vi "PM100D_Single_Value_ph.vi"(2 "Averaging Period (s)":dbl=1.0, 3 "Beam Name":string="Green Unshifted") -> (0 "Status":T1, 1 "Light Power mW":dbl=8.10606551e-08 format="%^#_9e")   [LabVIEW 2012]
doc: "This VI shows how to communicate with a PM100D optical power/energy meter with SCPI commands.\n- Initializing the instrument\n- Getting system info\n- Setting parameters\n- Measurement configuration\n- Measuring queue\n- Fetching and displaying a measurement value\n- Closing the application"
uses:
  Gen Trav/Multi_Run_Status.ctl
panel:
  out "error out":errorcluster
  out "Wavelength nm":string="488"
  out "IDN String":string="Thorlabs,PM100USB,P2000214,1.3.0\n"
  out "Sensor SN":string="10020635"
  out "Sensor Name":string="S121C"
  out "Sensor Flags":bool[](array[boolean])=[TRUE, FALSE, FALSE, FALSE, FALSE, TRUE, FALSE, FALSE, TRUE, FALSE, FALSE, FALSE, FALSE, FALSE, FALSE, FALSE, FALSE, FALSE, FALSE, FALSE, FALSE, FALSE, FALSE, FALSE, FALSE, FALSE, FALSE, FALSE, FALSE, FALSE, FALSE, FALSE]
  out "New":bool=TRUE
  out "Timeout [ms]":i32=3000
  in  "Readout Config":string(combo)="POW"
  out "Readout string":string="81.06nW"
  out "Error log":string
  out "Averaging Rate":i32=2000
  # "1 Power Sensor"
  # "2 Energy Sensor"
  # "4"
  # "8"
  # "16 Response settable"
  # "32 Wavelength settable"
  # "64 Tau (time constant) settable"
  # "128"
  # "256 With temperature sensor"
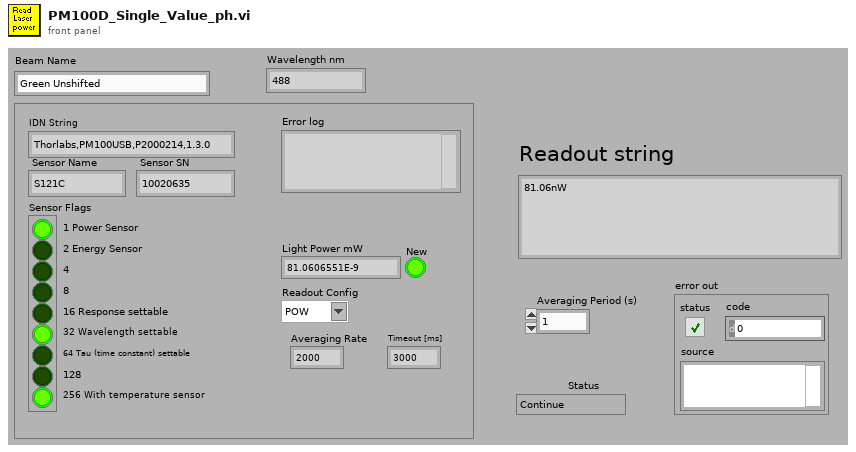
[diagram p1: front panel]
types:
  T1 = typedef "Multi_Run_Status.ctl" = enum16{"Continue", "Jump to Next Point", "Jump to Next Row", "Jump To Fall Back", "Terminate Run"}
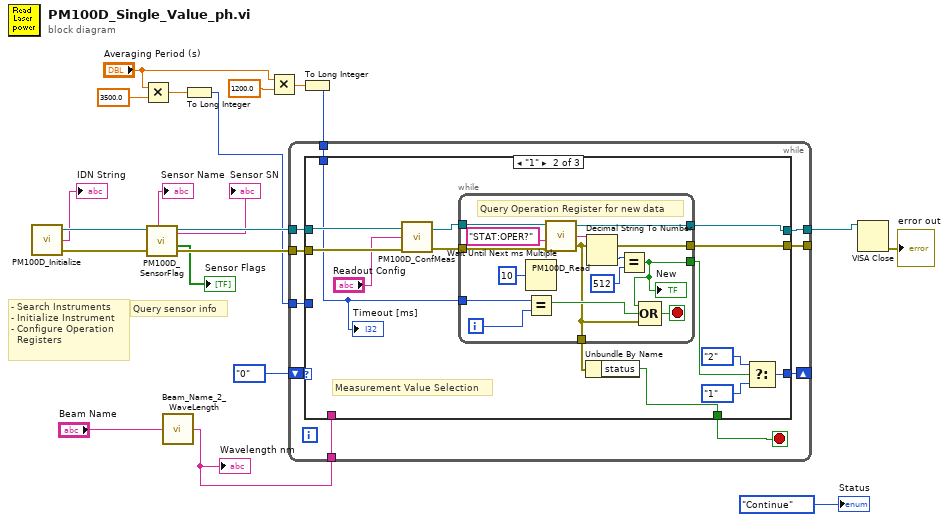
[diagram p0: block diagram]
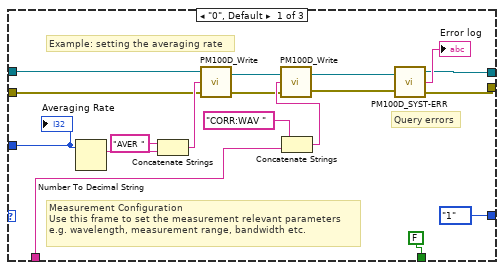
[diagram p2: hidden frame]
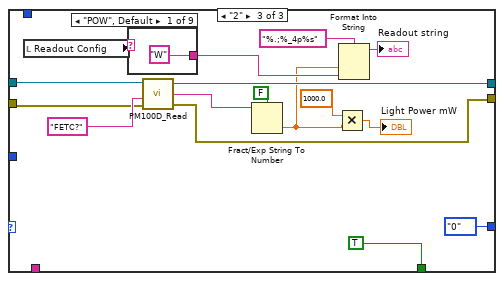
[diagram p3: hidden frame]
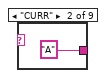
[diagram p4: hidden frame]
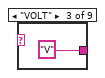
[diagram p5: hidden frame]
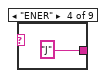
[diagram p6: hidden frame]
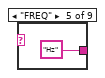
[diagram p7: hidden frame]
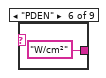
[diagram p8: hidden frame]
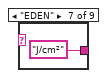
[diagram p9: hidden frame]
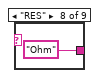
[diagram p10: hidden frame]
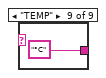
[diagram p11: hidden frame]
diagram:
  # "- Search Instruments\n- Initialize Instrument\n- Configure Operation\n  Registers"
  # "Query sensor info"
  n1 = call "PM100D_Initialize.vi"() -> ("error out"=w20:errorcluster, "Instrument"=→"IDN String":string, "VISA out"=w21:refnum<visa-resource-name>)  [unwired: 3 out]
  n2 = Multiply(x="Averaging Period (s)", y=3500.0) -> (x*y=w8:dbl)
  n3 = call "PM100D_SensorFlag.vi"("error in (no error)"=w20, "VISA in"=w21) -> ("error out"=w18:errorcluster, "flags"=→"Sensor Flags":bool[], "VISA out"=w19:refnum<visa-resource-name>, "sn"=→"Sensor SN":string, "name"=→"Sensor Name":string)  [unwired: 5 out]
  n4 = call "Beam_Name_2_WaveLength.vi"("Beam Name"="Beam Name") -> ("Wavelength nm"=w10:string)
  "Wavelength nm" <- w10
  n5 = To Long Integer(number=w8) -> (32bit integer=w7:i32)
  n6 = Multiply(x="Averaging Period (s)", y=1200.0) -> (x*y=w4:dbl)
  n7 = To Long Integer(number=w4) -> (32bit integer=w3:i32)
  n8 = while {
    tunnel: w19 -> [w31]
    tunnel: w18 -> [w30]
    shift-right: [w28] -> _
    shift-left: enum16{"0", "1", "2"}."0" -> [w29]
    tunnel: [w27] -> w2
    tunnel: [w26] -> _
    tunnel: w10 -> [w24]
    tunnel: w7 -> [w23]
    tunnel: w3 -> [w22]
    stop <- w25 stop-if-true
    n9 = case shown="\"1\"" w29 {
      tunnel: w31 -> [w47 w63 w91]
      tunnel: w30 -> [w44 w62 w90]
      tunnel: [enum16{"0", "1", "2"}."1" w57 enum16{"0", "1", "2"}."0"] -> w28
      tunnel: [w42 w59 w89] -> w27
      tunnel: [w41 w58 w82] -> w26
      tunnel: [FALSE w50 TRUE] -> w25
      tunnel: w24 -> [w37 _ _]
      tunnel: w23 -> [w32 _ _]
      tunnel: w22 -> [_ w52 _]
      frame "0", Default {
        # "Query errors"
        # "Example: setting the averaging rate"
        # "Measurement Configuration\nUse this frame to set the measurement relevant parameters\ne.g. wavelength, measurement range, bandwidth etc."
        n10 = Number To Decimal String(number=w32) -> (decimal integer string=w48:string)  [unwired: 1 out]
        n11 = Concatenate Strings("AVER " ("string"), w48) -> (w46:string)
        n12 = call "PM100D_Write.vi"("error in (no error)"=w44, "Command"=w46, "VISA in"=w47) -> ("error out"=w34:errorcluster, "VISA out"=w39:refnum<visa-resource-name>)
        n13 = Concatenate Strings("CORR:WAV " ("string"), w37) -> (w35:string)
        n14 = call "PM100D_Write.vi"("error in (no error)"=w34, "Command"=w35, "VISA in"=w39) -> ("error out"=w33:errorcluster, "VISA out"=w38:refnum<visa-resource-name>)
        n15 = call "PM100D_SYST-ERR.vi"("error out 2"=w33, "VISA In"=w38) -> ("error out"=w41:errorcluster, "Error"=→"Error log":string, "VISA Out"=w42:refnum<visa-resource-name>)  [unwired: 1 out]
        "Averaging Rate" <- w32
      }
      frame "1" {
        # "Measurement Value Selection"
        n16 = call "PM100D_ConfMeas.vi"("error in"=w62, "Conf:"="Readout Config", "VISA In"=w63) -> ("error out"=w60:errorcluster, "dup VISA session"=w61:refnum<visa-resource-name>)
        n17 = while {
          tunnel: w61 -> [w73]
          tunnel: w60 -> [w72]
          tunnel: [w71] -> w59
          tunnel: [w64] -> w58
          tunnel: [w67] -> w54
          tunnel: w52 -> [w66]
          tunnel: [w64] -> w51
          i -> [w69]
          stop <- w70 stop-if-true
          # "Query Operation Register for new data"
          n18 = Wait Until Next ms Multiple(millisecond multiple=u32 10) -> ()  [unwired: 1 out]
          n19 = Equal?(x=w66, y=w69) -> (x = y?=w68:bool)
          n20 = call "PM100D_Read.vi"("error in (no error)"=w72, "Command"="STAT:OPER?", "VISA in"=w73) -> ("error out"=w64:errorcluster, "ReadValue"=w76:string, "VISA out"=w71:refnum<visa-resource-name>)  [unwired: 1 out]
          n21 = Decimal String To Number(string=w76) -> (number=w75:i32)  [unwired: 1 in, 2 out]
          n22 = Equal?(x=w75, y=512) -> (x = y?=w67:bool)
          "New" <- w67
          n23 = Compound Arithmetic op=OR(w67, w68, w64) -> (w70:bool)
        }
        n24 = Unbundle By Name(w51) -> ("status"=w50:bool)
        n25 = Select(t=enum16{"0", "1", "2"}."2", s=w54, f=enum16{"0", "1", "2"}."1") -> (s? t:f=w57:enum16{"0", "1", "2"})
        "Timeout [ms]" <- w52
      }
      frame "2" {
        n26 = local read "Readout Config"() -> (w88:string)
        n27 = case shown="\"POW\", Default" w88 {
          tunnel: ["W" "A" "V" "J" "Hz" "W/cm²" "J/cm²" "Ohm" "°C"] -> w84
          frame "POW", Default {
          }
          frame "CURR" {
          }
          frame "VOLT" {
          }
          frame "ENER" {
          }
          frame "FREQ" {
          }
          frame "PDEN" {
          }
          frame "EDEN" {
          }
          frame "RES" {
          }
          frame "TEMP" {
          }
        }
        n28 = call "PM100D_Read.vi"("error in (no error)"=w90, "Command"="FETC?", "VISA in"=w91) -> ("error out"=w82:errorcluster, "ReadValue"=w87:string, "VISA out"=w89:refnum<visa-resource-name>)  [unwired: 1 out]
        n29 = Fract/Exp String To Number(use system decimal point (T)=FALSE, string=w87) -> (number=w79:dbl)  [unwired: 3 out]
        n30 = Multiply(x=1000.0, y=w79) -> (x*y=→"Light Power mW":dbl)
        n31 = Format Into String(format string="%.;%_4p%s", w79, w84) -> (resulting string=→"Readout string":string)  [unwired: 2 in, 1 out]
      }
    }
  }
  n32 = VISA Close(VISA resource name=w2) -> (error out=→"error out":errorcluster)  [unwired: 1 in]
  "Status" <- Multi_Run_Status."Continue" ("Status")
